vi "Correct funct acq lengths.vi"(8 "error in (no error)":errorcluster, 11 "Cool-down time (s)":refnum<vi>) -> (0 "error out":errorcluster, 2 "Cool-down time (s)":dbl, 3 "Cool-down time (s)":refnum<vi>)   [LabVIEW 2013]
uses:
  Typedefs/ROI management FG states.ctl
  User Interface/ROI Entry screen/Globals/gl_ROI Entry UI globals.vi
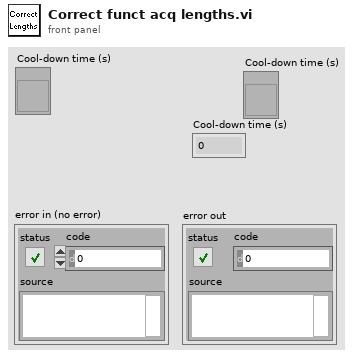
[diagram p1: front panel]
types:
  T1 = typedef "ROI management FG states.ctl" = enum16{"Read", "Write", "Clear Last", "Clear All", "Update ROIs time", "Reload last ROI set", "Offset all ROI", "Offset visible ROI"}
  T2 = typedef "ROI entry screen ctrl refs cluster.ctl" = cluster{"Done button":refnum<vi>, "Imaging button":refnum<vi>, "Acquisition button":refnum<vi>, "POI dwell time (us)":refnum<vi>, "Scan dwell time per pixel (us)":refnum<vi>, "# of planes":refnum<vi>, "Zoom":refnum<vi>, "Equal size":refnum<vi>, "Channel":refnum<vi>, "Image Display":refnum<vi>, "Z-Plane Selector":refnum<vi>, "Number of lines left":refnum<vi>, "Z-stack folder path":refnum<vi>, "POI Density":refnum<vi>, "Arb Plane Entry":refnum<vi>, "Whole plane":refnum<vi>, "Clear Last":refnum<vi>, "Clear All":refnum<vi>, "Trial Length (sec)":refnum<vi>, "Palette Type":refnum<vi>, "Intensity slider":refnum<vi>, "# POI":refnum<vi>, "Max Z Proj":refnum<vi>, "Zplane ind":refnum<vi>, "Wavelength (nm)":refnum<vi>, "Number of Trials":refnum<vi>, "Funct stim.trig.enable":refnum<vi>, "Funct stim.trig.delay (s)":refnum<vi>, "Line Mode":refnum<vi>, "Step size (µm)":refnum<vi>, "ROI move mode":refnum<vi>, "Cool-down time (s)":refnum<vi>, "Enable cool-down time":refnum<vi>, "Motor Z ind. (um)":refnum<vi>, "AOL Z ind. (um)":refnum<vi>}
  T3 = typedef "ROI parameters data type.ctl" = cluster{"ROI index":dbl, "ROI ID":dbl, "ROI Time (ns)":dbl, "Pixels in ROI":dbl, "X start":dbl, "Y start":dbl, "Z start":dbl, "X stop":dbl, "Y stop":dbl, "Z stop":dbl, "Angle (deg)":dbl, "Composite ID":dbl, "Number of lines":dbl, "Frame Size":dbl, "Zoom":dbl, "Laser Power (%)":dbl, "ROI group ID":dbl}
  T4 = typedef "AOL_Globals.ctl" = cluster{"Imaging Protocol":T5, "Number of POI":u16, "Number of Miniscans":u16, "Number of Trials":u16, "Number of Cycles ":u64, "# Averaged Frames":u16, "Laser power (%)":u8, "Pockels":dbl, "Acquisition Length (sec)":dbl, "Fill time (us)":dbl, "POI Dwell time (us)":dbl, "Miniscan Dwell time per pixel (us)":dbl, "PMT 1":dbl, "PMT 2":dbl, "Back Apperture":dbl, "Frame Size":T6, "Center Frequency":dbl, "Field of View":dbl, "DwellTime (us)":dbl, "Wavelength (nm)":dbl, "Zoom":dbl, "AOL Z":dbl, "AOL Mode":T7, "GridXY":dbl, "GridZ":dbl, "TriggerPeriod (sec)":dbl, "Number of Pixels in Miniscan":u16, "Experiment folder path":path, "X centre":dbl, "Y centre":dbl, "Angle (degrees)":dbl, "Plane Mode":T8, "Threshold":u16[], "Regenerate Chirps":bool, "Rectangle ROI length (pixels)":u16, "Rectangle ROI height (pixels)":u16, "AOD fill":u16, "Samples Wait after Trigger":u16, "StartUp Delay":i32, "Slip Cycle":u32, "Add Cycle":bool}
  T5 = typedef "Imaging Protocols enum.ctl" = enum16{"AOL Z-Stack", "Motor Z Stack", "Functional Acquisition", "Single Plane Acquisition", "Volume Acquisition", "Live Imaging", "Live Plane Imaging", "Live Volume Imaging"}
  T6 = typedef "Frame Size.ctl" = u16
  T7 = typedef "AOL modes.ctl" = enum16{"Raster", "Structural", "Pointing", "Mini Scan", "Alignment"}
  T8 = typedef "Plane Mode.ctl" = u16
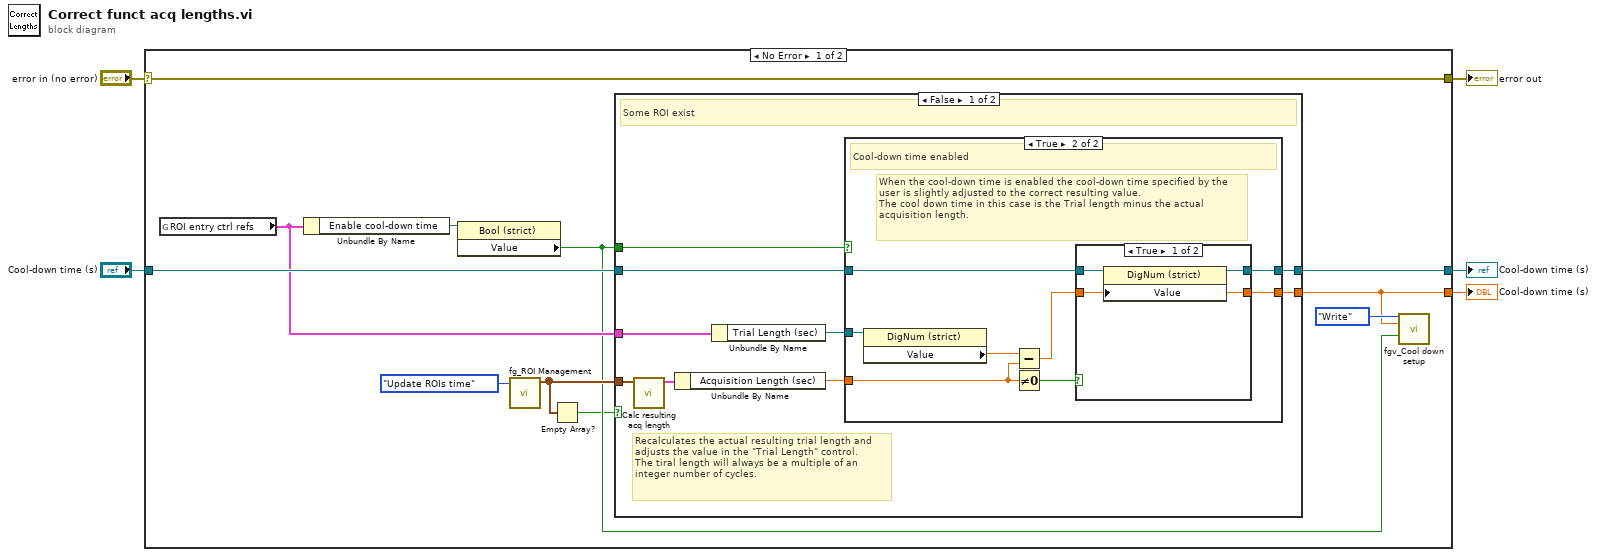
[diagram p0: block diagram]
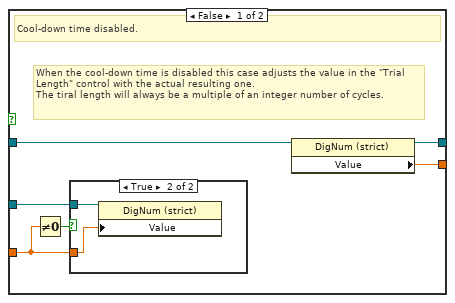
[diagram p2: hidden frame]
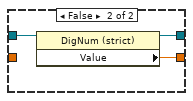
[diagram p4: hidden frame]
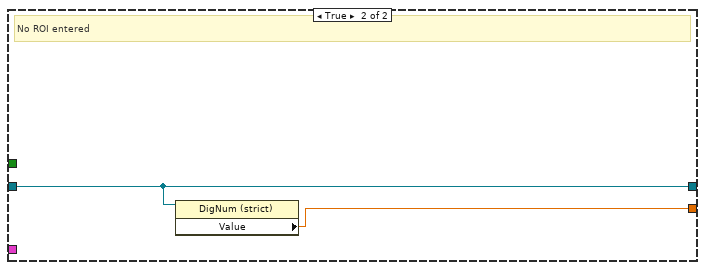
[diagram p5: hidden frame]
diagram:
  n1 = case shown="No Error" "error in (no error)" {
    selector: "error in (no error)" -> [w14 w51]
    tunnel: [w14 w51] -> w5
    tunnel: "Cool-down time (s)" -> [w16 w50]
    tunnel: [w10 _] -> w2
    tunnel: [w15 w50] -> w1
    frame No Error {
      n2 = global read "gl_ROI Entry UI globals.vi" "ROI entry ctrl refs"() -> (w8:T2)
      n3 = Unbundle By Name(w8) -> ("Enable cool-down time"=w9:refnum<vi>)
      n4 = property on="Property Node" class="Bool (strict)"(reference=w9) -> ("Value"=w7:bool)  [unwired: 1 in, 2 out]
      n5 = call "fg_ROI Management.vi"("Function"=ROI_management_FG_states."Update ROIs time") -> ("ROI Setup"=w12:T3[])  [unwired: 6 in, 4 out]
      n6 = Empty Array?(array=w12) -> (empty?=w6:bool)
      n7 = case shown="False" w6 {
        tunnel: w16 -> [w25 w49]
        tunnel: [w24 w48] -> w10
        tunnel: [w23 w49] -> w15
        tunnel: w12 -> [w22 _]
        tunnel: w7 -> [w18 _]
        tunnel: w8 -> [w17 _]
        frame False {
          # "Recalculates the actual resulting trial length and adjusts the value in the \"Trial Length\" control.\nThe tiral length will always be a multiple of an integer number of cycles."
          # "Some ROI exist"
          n8 = call "Calc resulting acq length.vi"("XYZ_Coordinates"=w22) -> ("Output cluster"=w21:T4)  [unwired: 9 in, 1 out]
          n9 = Unbundle By Name(w21) -> ("Acquisition Length (sec)"=w20:dbl)
          n10 = Unbundle By Name(w17) -> ("Trial Length (sec)"=w19:refnum<vi>)
          n11 = case shown="True" w18 {
            tunnel: w25 -> [w29 w41]
            tunnel: [w30 w40] -> w23
            tunnel: [w28 w34] -> w24
            tunnel: w20 -> [w26 w36]
            tunnel: w19 -> [w31 w38]
            frame False {
              # "When the cool-down time is disabled this case adjusts the value in the \"Trial Length\" control with the actual resulting one.\nThe tiral length will always be a multiple of an integer number of cycles."
              # "Cool-down time disabled."
              n12 = Not Equal To 0?(x=w26) -> (x != 0?=w27:bool)
              n13 = case shown="True" w27 {
                tunnel: w26 -> [_ w33]
                tunnel: w31 -> [_ w32]
                frame False {
                }
                frame True {
                  n14 = property on="Property Node" class="DigNum (strict)"(reference=w32, "Value"=w33) -> ()  [unwired: 1 in, 2 out]
                }
              }
              n15 = property on="Property Node" class="DigNum (strict)"(reference=w29) -> (reference out=w30:refnum<vi>, "Value"=w28:dbl)  [unwired: 1 in, 1 out]
            }
            frame True {
              # "When the cool-down time is enabled the cool-down time specified by the user is slightly adjusted to the correct resulting value.\nThe cool down time in this case is the Trial length minus the actual acquisition length."
              # "Cool-down time enabled"
              n16 = property on="Property Node" class="DigNum (strict)"(reference=w38) -> ("Value"=w39:dbl)  [unwired: 1 in, 2 out]
              n17 = Subtract(x=w39, y=w36) -> (x-y=w37:dbl)
              n18 = Not Equal To 0?(x=w36) -> (x != 0?=w35:bool)
              n19 = case shown="True" w35 {
                tunnel: w41 -> [w44 w47]
                tunnel: [w43 w46] -> w40
                tunnel: w37 -> [w42 _]
                tunnel: [w42 w45] -> w34
                frame True {
                  n20 = property on="Property Node" class="DigNum (strict)"(reference=w44, "Value"=w42) -> (reference out=w43:refnum<vi>)  [unwired: 1 in, 1 out]
                }
                frame False {
                  n21 = property on="Property Node" class="DigNum (strict)"(reference=w47) -> (reference out=w46:refnum<vi>, "Value"=w45:dbl)  [unwired: 1 in, 1 out]
                }
              }
            }
          }
        }
        frame True {
          # "No ROI entered"
          n22 = property on="Property Node" class="DigNum (strict)"(reference=w49) -> ("Value"=w48:dbl)  [unwired: 1 in, 2 out]
        }
      }
      n23 = call "fgv_Cool down setup.vi"("Function"=enum16{"Intialize", "Write", "Read", "Clear"}."Write", "Cool-down time (s)"=w10, "Enable cool-down time"=w7) -> ()  [unwired: 10 in, 3 out]
    }
    frame Error {
    }
  }
  "error out" <- w5
  "Cool-down time (s)" <- w1
  "Cool-down time (s)" <- w2
